vi "SubVI_WaitTrigger.vi"() -> (0 "error out":errorcluster caption="에러 출력", 3 "data":bool caption="데이터")   [LabVIEW 2016]
uses:
  Ctrls/exit.ctl
  <vilib>/DAQmx/read.llb/DAQmx Read (Digital Bool 1Line 1Point).vi
  <vilib>/DAQmx/create/channels.llb/DAQmx Create Channel (DI-Digital Input).vi
  <vilib>/DAQmx/miscellaneous.llb/DAQmx Fill In Error Info.vi
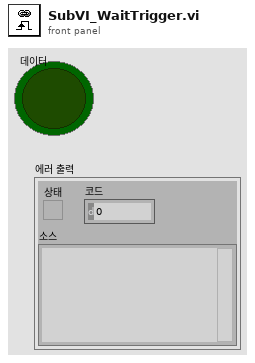
[diagram p1: front panel]
types:
  T1 = typedef "exit.ctl" = enum16{"default", "ini", "exit"}
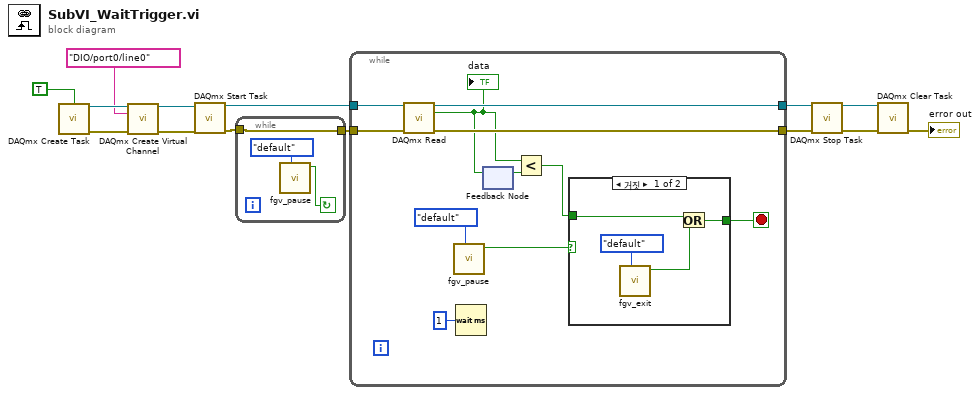
[diagram p0: block diagram]
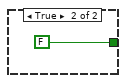
[diagram p2: hidden frame]
diagram:
  n1 = call <vilib>:"DAQmx Create Task.vi"("auto cleanup"=TRUE) -> ("task out"=w13:refnum<k21>, "error out"=w3:errorcluster)  [unwired: 13 in]
  n2 = call-poly <vilib>:"DAQmx Create Virtual Channel.vi"("task in"=w13, "lines"=tag "DIO/port0/line0", "error in"=w3) -> ("task out"=w4:refnum<k21>, "error out"=w5:errorcluster)  [unwired: 11 in]
  n3 = call <vilib>:"DAQmx Start Task.vi"("task/channels in"=w4, "error in"=w5) -> ("task out"=w11:refnum<k21>, "error out"=w1:errorcluster)  [unwired: 12 in]
  n4 = while {
    tunnel: [w15] -> w2
    tunnel: w1 -> [w15]
    stop <- w16 continue-if-true
    n5 = call "fgv_pause.vi"("cmd"=enum16{"default", "ini", "pause"}."default") -> ("pause"=w16:bool)  [unwired: 9 in, 1 out]
  }
  n6 = while {
    tunnel: w11 -> [w28]
    tunnel: w2 -> [w27]
    tunnel: [w24] -> w9
    tunnel: [w26] -> w8
    stop <- w25 stop-if-true
    n7 = call-poly <vilib>:"DAQmx Read.vi"("task/channels in"=w28, "error in"=w27) -> ("task out"=w26:refnum<k21>, "data"=w19:bool, "error out"=w24:errorcluster)  [unwired: 11 in]
    "data" <- w19
    n8 = call "fgv_pause.vi"("cmd"=enum16{"default", "ini", "pause"}."default") -> ("pause"=w22:bool)  [unwired: 9 in, 1 out]
    n9 = Wait (ms)(milliseconds to wait=u32 1 ("대기 시간(ms)")) -> ()  [unwired: 1 out]
    n10 = feedback-in #1(w19) -> ()
    n11 = feedback #1() -> (w20:bool)  [unwired: 1 in]
    n12 = Less?(x=w19, y=w20) -> (x < y?=w18:bool)
    n13 = case shown="거짓" w22 {
      tunnel: [w32 FALSE] -> w25
      tunnel: w18 -> [w31 _]
      frame False {
        n14 = call "fgv_exit.vi"("cmd"=exit."default") -> ("stop"=w29:bool)  [unwired: 9 in, 1 out]
        n15 = Or(x=w31, y=w29) -> (x .or. y?=w32:bool)
      }
      frame True {
      }
    }
  }
  n16 = call <vilib>:"DAQmx Stop Task.vi"("task/channels in"=w8, "error in"=w9) -> ("task out"=w10:refnum<k21>, "error out"=w7:errorcluster)  [unwired: 12 in]
  n17 = call <vilib>:"DAQmx Clear Task.vi"("task in"=w10, "error in"=w7) -> ("error out"=→"error out":errorcluster)  [unwired: 13 in]
